vi "TDMS读取.vi"() -> ()   [LabVIEW 2017]
panel:
  out "组名称输出 2":string
  out "通道名称输出 2":string[](array[string])
  out "通道名称输出":string[](array[string])
  out "组名称输出":string
  out "波形图":waveform(dbl)[](graph)
  in  "错误输入（无错误）":errorcluster
  in  "路径":path
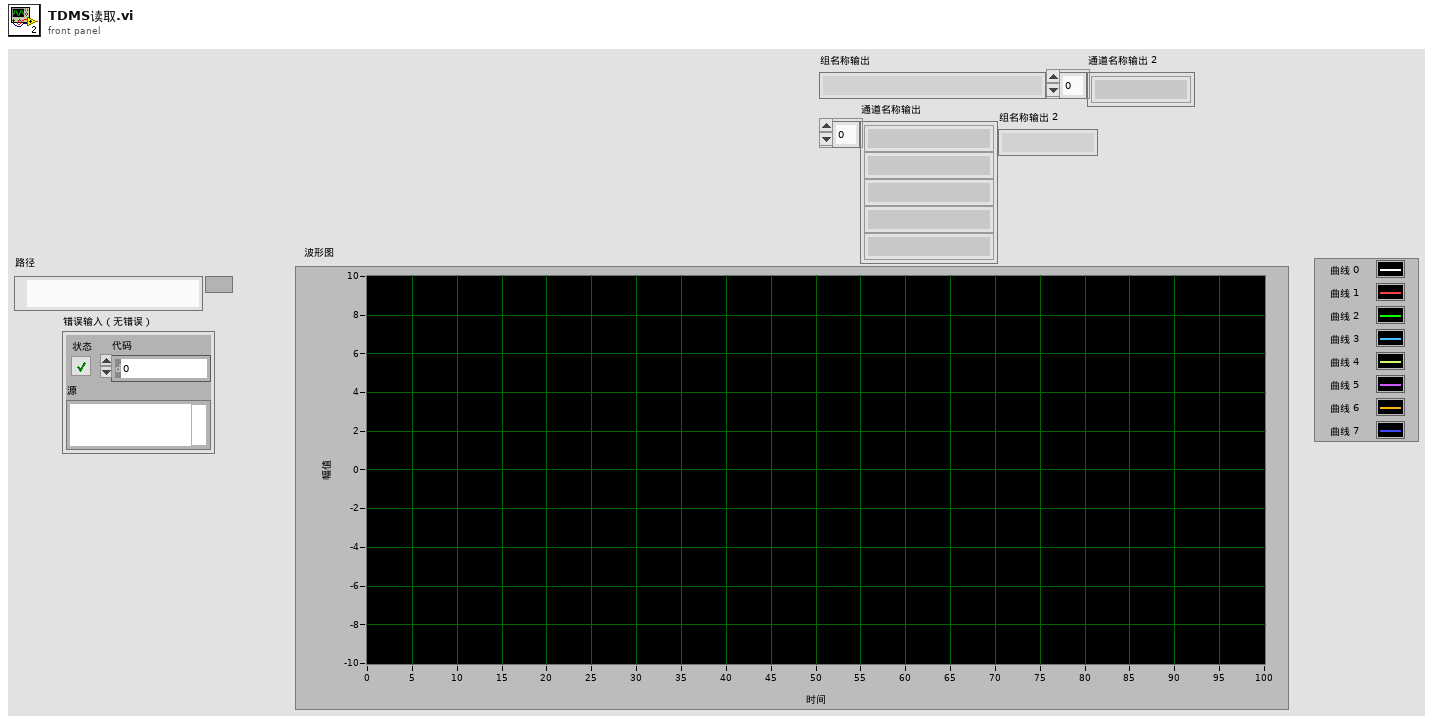
[diagram p1: front panel]
types:
  T1 = enum16{"open", "open or create", "create or replace", "create", "open (read-only)"}
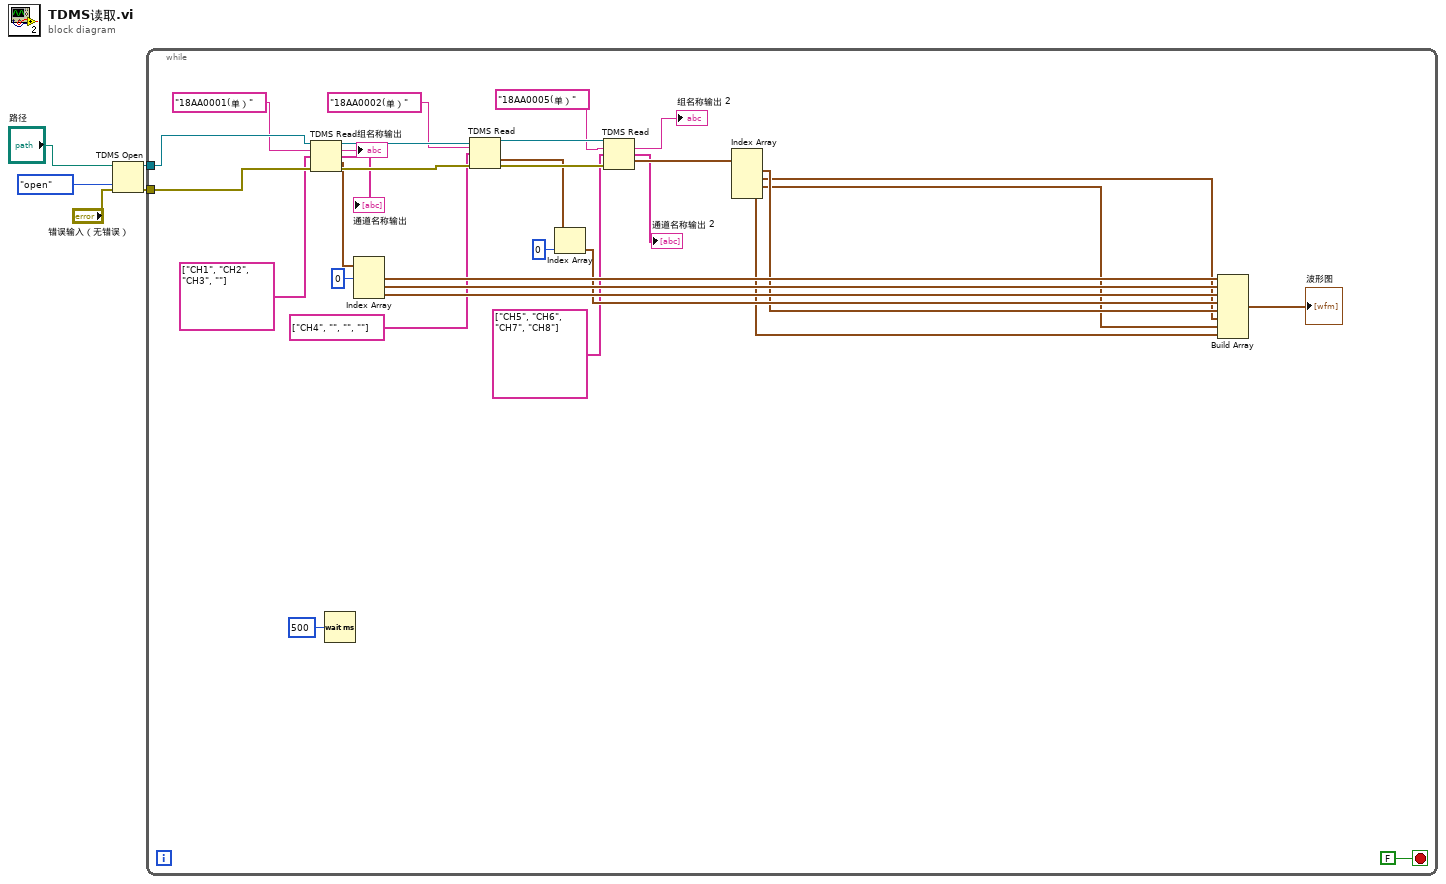
[diagram p0: block diagram]
diagram:
  n1 = TDMS Open(8:"错误输入（无错误）", 10:T1."open" ("操作(0:open)"), 11:"路径") -> (0:w2:errorcluster, 3:w1:refnum<k34>)  [unwired: 4 in]
  n2 = while {
    tunnel: w2 -> [w30]
    tunnel: w1 -> [w33]
    stop <- FALSE stop-if-true
    n3 = TDMS Read(0:w33, 5:"18AA0001(单）" ("组名称输入"), 7:string[] ["CH1", "CH2", "CH3", ""], 11:w30) -> (4:w37:refnum<k34>, 6:→"组名称输出":string, 8:→"通道名称输出":string[], 10:w29:waveform(dbl)[], 15:w35:errorcluster)  [unwired: 4 in, 1 out]
    n4 = Wait (ms)(milliseconds to wait=u32 500 ("等待时间（毫秒）")) -> ()  [unwired: 1 out]
    n5 = Index Array(array=w29, index #1=0 ("索引")) -> (element #1=w27:waveform(dbl), element #2=w26:waveform(dbl), element #3=w25:waveform(dbl))  [unwired: 2 in]
    n6 = TDMS Read(0:w37, 5:"18AA0002(单）" ("组名称输入"), 7:string[] ["CH4", "", "", ""], 11:w35) -> (4:w36:refnum<k34>, 10:w22:waveform(dbl)[], 15:w34:errorcluster)  [unwired: 4 in, 3 out]
    n7 = Index Array(array=w22, index=0 ("索引")) -> (element=w20:waveform(dbl))
    n8 = TDMS Read(0:w36, 5:"18AA0005(单）" ("组名称输入"), 7:string[] ["CH5", "CH6", "CH7", "CH8"], 11:w34) -> (6:→"组名称输出 2":string, 8:→"通道名称输出 2":string[], 10:w24:waveform(dbl)[])  [unwired: 4 in, 3 out]
    n9 = Index Array(array=w24) -> (element #1=w19:waveform(dbl), element #2=w18:waveform(dbl), element #3=w17:waveform(dbl), element #4=w16:waveform(dbl))  [unwired: 4 in]
    n10 = Build Array(w27, w26, w25, w20, w19, w18, w17, w16) -> (→"波形图":waveform(dbl)[])
  }
